vi "IVIDMM-Synchronized-Readout.vi"() -> ()   [LabVIEW 2015, in "IVI_DMM.lvlib"]
uses:
  IVI_DMM.lvlib
panel:
  in  "IVI Logical Names":refnum<k15>[](array[refnum])=["DMM3458A_GPIB0_21", "DMM3458A_GPIB0_22"]
  out "dt":dbl[unit] format="%.3f"
  out "Apertures":dbl[unit][](array[numeric])
  out "Samples":i32[](array[numeric])
  out "Graph":dbl[unit][](graph)
  in  "sample count":i32=10 caption="sample count (1)"
  in  "sample interval":dbl[unit]=0.1 caption="sample interval (0.0 s)" format="%.3f"
  out "error out":errorcluster
  in  "Stop":bool
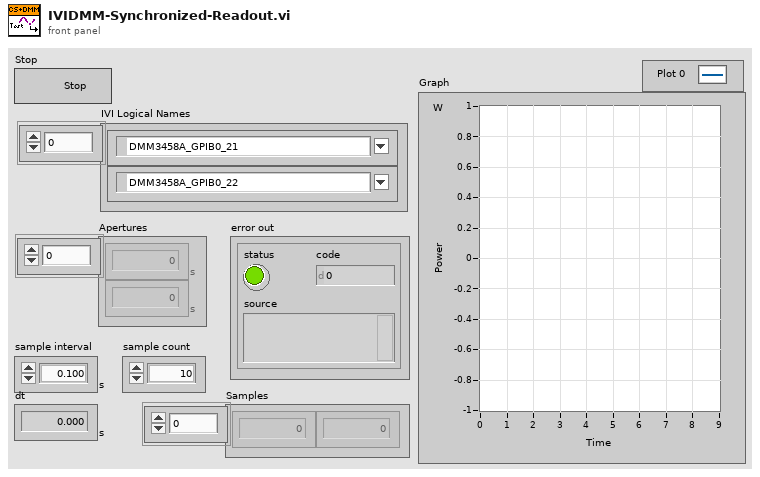
[diagram p1: front panel]
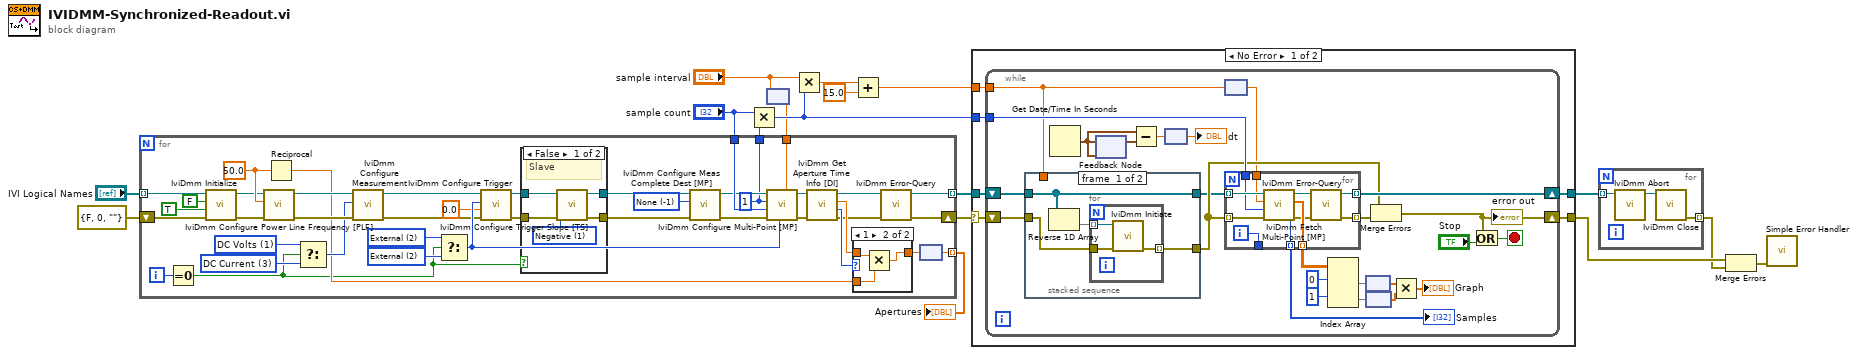
[diagram p0: block diagram]
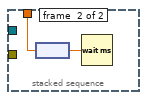
[diagram p2: hidden frame]
diagram:
  n1 = node("sample interval") -> (w3:dbl)
  n2 = for {
    tunnel: [w18] -> w17 mode=indexing
    shift-right: [w20] -> w16
    shift-left: errorcluster {"status"=FALSE, "code"=0, "source"=""} ("error out") -> [w26]
    tunnel: "sample count" -> [w48]
    tunnel: w3 -> [w47]
    tunnel: [w41] -> w8 mode=indexing
    tunnel: [w27] -> w7
    tunnel: "IVI Logical Names" -> [w24] mode=indexing
    i -> [w52]
    w49 = -1 items=["None"=-1, "External"=2, "PXI TRIG0 or VXI TTL0"=111, "PXI TRIG1 or VXI TTL1"=112, "PXI TRIG2 or VXI TTL2"=113, "PXI TRIG3 or VXI TTL3"=114, "PXI TRIG4 or VXI TTL4"=115, "PXI TRIG5 or VXI TTL5"=116, "PXI TRIG6 or VXI TTL6"=117, "PXI TRIG7 or VXI TTL7"=118, "ECL0"=119, "ECL1"=120, "PXI Star"=131, "RTSI 0"=140, "RTSI 1"=141, "RTSI 2"=142, "RTSI 3"=143, "RTSI 4"=144, "RTSI 5"=145, "RTSI 6"=146] ("meas complete dest (None)")
    w50 = 2 items=["Immediate"=1, "External"=2, "Software Trigger Function"=3, "Interval"=10, "PXI TRIG0 or VXI TTL0"=111, "PXI TRIG1 or VXI TTL1"=112, "PXI TRIG2 or VXI TTL2"=113, "PXI TRIG3 or VXI TTL3"=114, "PXI TRIG4 or VXI TTL4"=115, "PXI TRIG5 or VXI TTL5"=116, "PXI TRIG6 or VXI TTL6"=117, "PXI TRIG7 or VXI TTL7"=118, "ECL0"=119, "ECL1"=120, "PXI Star"=131, "RTSI 0"=140, "RTSI 1"=141, "RTSI 2"=142, "RTSI 3"=143, "RTSI 4"=144, "RTSI 5"=145, "RTSI 6"=146] ("sample trigger (Immediate)")
    w51 = 2 items=["Immediate"=1, "External"=2, "Software Trigger Function"=3, "Interval"=10, "PXI TRIG0 or VXI TTL0"=111, "PXI TRIG1 or VXI TTL1"=112, "PXI TRIG2 or VXI TTL2"=113, "PXI TRIG3 or VXI TTL3"=114, "PXI TRIG4 or VXI TTL4"=115, "PXI TRIG5 or VXI TTL5"=116, "PXI TRIG6 or VXI TTL6"=117, "PXI TRIG7 or VXI TTL7"=118, "ECL0"=119, "ECL1"=120, "PXI Star"=131, "RTSI 0"=140, "RTSI 1"=141, "RTSI 2"=142, "RTSI 3"=143, "RTSI 4"=144, "RTSI 5"=145, "RTSI 6"=146] ("sample trigger (Immediate)")
    w27 = 1 ("trigger count (1)")
    w53 = 3 items=["DC Volts"=1, "AC Volts"=2, "DC Current"=3, "AC Current"=4, "2 Wire Resistance"=5, "4 Wire Resistance"=101, "AC + DC Volts"=106, "AC + DC Current"=107, "Frequency"=104, "Period"=105, "Temperature"=108] ("measurement function (DC Volts)")
    w55 = 1 items=["DC Volts"=1, "AC Volts"=2, "DC Current"=3, "AC Current"=4, "2 Wire Resistance"=5, "4 Wire Resistance"=101, "AC + DC Volts"=106, "AC + DC Current"=107, "Frequency"=104, "Period"=105, "Temperature"=108] ("measurement function (DC Volts)")
    w43 = 50.0 ("power line frequency (60.0 Hz)")
    n3 = Equal To 0?(x=w52) -> (x = 0?=w38:bool)
    n4 = call <vilib>:"IviDmm Initialize.vi"("error in (no error)"=w26, "reset device (True)"=TRUE ("Reset (F)"), "id query (True)"=FALSE, "logical name (\"SampleDmm\")"=w24) -> ("error out"=w22:errorcluster, "instrument handle out"=w23:refnum<k15>)  [unwired: 6 in]
    n5 = call <vilib>:"IviDmm Configure Power Line Frequency [PLF].vi"("error in (no error)"=w22, "power line frequency (60.0 Hz)"=w43, "instrument handle"=w23) -> ("error out"=w56:errorcluster, "instrument handle out"=w57:refnum<k15>)  [unwired: 7 in]
    n6 = Reciprocal(x=w43) -> (1/x=w42:dbl)
    n7 = Select(t=w55, s=w38, f=w53) -> (s? t:f=w54:i32)
    n8 = call <vilib>:"IviDmm Configure Measurement.vi"("error in (no error)"=w56, "measurement function (DC Volts)"=w54, "instrument handle"=w57) -> ("error out"=w32:errorcluster, "instrument handle out"=w33:refnum<k15>)  [unwired: 7 in]
    n9 = Select(t=w51, s=w38, f=w50) -> (s? t:f=w35:i32)
    n10 = call <vilib>:"IviDmm Configure Trigger.vi"("error in (no error)"=w32, "trigger delay (0.0 s)"=0.0, "trigger source (Immediate)"=w35, "instrument handle"=w33) -> ("error out"=w36:errorcluster, "instrument handle out"=w37:refnum<k15>)  [unwired: 6 in]
    n11 = case shown="False" w38 {
      tunnel: w37 -> [w63 w65]
      tunnel: [w62 w65] -> w40
      tunnel: w36 -> [w61 w64]
      tunnel: [w60 w64] -> w39
      frame False {
        w59 = 1 items=["Positive", "Negative"] ("trigger slope (0: Positive)")
        # "Slave"
        n12 = call <vilib>:"IviDmm Configure Trigger Slope [TS].vi"("error in (no error)"=w61, "trigger slope (0: Positive)"=w59, "instrument handle"=w63) -> ("error out"=w60:errorcluster, "instrument handle out"=w62:refnum<k15>)  [unwired: 7 in]
      }
      frame True {
        # "Master"
      }
    }
    n13 = call <vilib>:"IviDmm Configure Meas Complete Dest [MP].vi"("error in (no error)"=w39, "meas complete dest (None)"=w49, "instrument handle"=w40) -> ("error out"=w30:errorcluster, "instrument handle out"=w31:refnum<k15>)  [unwired: 7 in]
    n14 = call <vilib>:"IviDmm Configure Multi-Point [MP].vi"("sample interval (0.0 s)"=w47, "sample trigger (Immediate)"=w35, "error in (no error)"=w30, "sample count (1)"=w48, "trigger count (1)"=w27, "instrument handle"=w31) -> ("error out"=w28:errorcluster, "instrument handle out"=w29:refnum<k15>)  [unwired: 4 in]
    n15 = call <vilib>:"IviDmm Get Aperture Time Info [DI].vi"("error in (no error)"=w28, "instrument handle"=w29) -> ("error out"=w21:errorcluster, "aperture time units"=w46:i32, "aperture time (sec)"=w45:dbl, "instrument handle out"=w19:refnum<k15>)  [unwired: 6 in]
    n16 = case shown="1" w46 {
      tunnel: w45 -> [w66 w69]
      tunnel: [w66 w67] -> w44
      tunnel: w42 -> [_ w68]
      frame 0, Default {
      }
      frame 1 {
        n17 = Multiply(x=w69, y=w68) -> (x*y=w67:dbl)
      }
    }
    n18 = call <vilib>:"IviDmm Error-Query.vi"("error in (no error)"=w21, "instrument handle"=w19) -> ("error out"=w20:errorcluster, "instrument handle out"=w18:refnum<k15>)  [unwired: 6 in, 2 out]
    n19 = node(w44) -> (w41:dbl[unit])
  }
  "Apertures" <- w8
  n20 = Multiply(x="sample count", y=w7) -> (x*y=w5:i32)
  n21 = Multiply(x="sample interval", y=w5) -> (x*y=w11:dbl[unit])
  n22 = Add(x=w11, y=dbl[unit] 15.0 ("x")) -> (x+y=w9:dbl[unit])
  n23 = case shown="No Error" w16 {
    selector: w16 -> [w74 w121]
    tunnel: w17 -> [w75 w122]
    tunnel: [w73 w122] -> w15
    tunnel: [w72 w121] -> w14
    tunnel: w9 -> [w71 _]
    tunnel: w5 -> [w70 _]
    frame No Error {
      n24 = while {
        shift-right: [w82] -> w72
        shift-left: w74 -> [w100]
        shift-right: [w98] -> w73
        shift-left: w75 -> [w97]
        tunnel: w71 -> [w77]
        tunnel: w70 -> [w96]
        stop <- w89 stop-if-true
        n25 = stacked-sequence {
          tunnel: w100 -> [w104 _]
          tunnel: w97 -> [w103 _]
          tunnel: [w101 _] -> w81
          tunnel: w77 -> [_ w108]
          tunnel: [w103 _] -> w76
          frame #0 {
            n26 = Reverse 1D Array(array=w103) -> (reversed array=w102:refnum<k15>[])
            n27 = for {
              tunnel: w102 -> [w105] mode=indexing
              tunnel: w104 -> [w107]
              tunnel: [w106] -> w101 mode=indexing
              n28 = call <vilib>:"IviDmm Initiate.vi"("error in (no error)"=w107, "instrument handle"=w105) -> ("error out"=w106:errorcluster)  [unwired: 8 in, 1 out]
            }
          }
          frame #1 {
            n29 = node(w108) -> (w109:dbl)
            n30 = Wait (ms)(milliseconds to wait=w109) -> ()  [unwired: 1 out]
          }
        }
        n31 = Get Date/Time In Seconds() -> (seconds since 1Jan1904=w86:timestamp)
        n32 = feedback #1(w86) -> (w85:timestamp)
        n33 = feedback-in #1(w86) -> ()
        n34 = Subtract(x=w86, y=w85) -> (x-y=w84:dbl)
        n35 = node(w84) -> (→"dt":dbl[unit])
        n36 = node(w77) -> (w78:dbl)
        n37 = for {
          tunnel: w76 -> [w119] mode=indexing
          tunnel: [w112] -> w98 mode=indexing
          tunnel: [w120] -> _
          tunnel: w96 -> [w117]
          tunnel: [w116] -> w95 mode=indexing
          tunnel: [w115] -> w87 mode=indexing
          tunnel: w78 -> [w113]
          tunnel: [w111] -> w88 mode=indexing
          tunnel: w81 -> [w114] mode=indexing
          i -> [w120]
          n38 = call <vilib>:"IviDmm Fetch Multi-Point [MP].vi"("error in (no error)"=w114, "array size (1)"=w117, "maximum time (5000 ms)"=w113, "instrument handle"=w119) -> ("error out"=w110:errorcluster, "actual number of points"=w115:i32, "reading array"=w116:dbl[], "instrument handle out"=w118:refnum<k15>)  [unwired: 4 in]
          n39 = call <vilib>:"IviDmm Error-Query.vi"("error in (no error)"=w110, "instrument handle"=w118) -> ("error out"=w111:errorcluster, "instrument handle out"=w112:refnum<k15>)  [unwired: 6 in, 2 out]
        }
        "Samples" <- w87
        n40 = Index Array(array=w95, index (row) #1=0 ("index (row)"), index (row) #2=1 ("index (row)")) -> (element #1=w92:dbl[], element #2=w91:dbl[])  [unwired: 2 in]
        n41 = node(w92) -> (w80:dbl[unit][])
        n42 = node(w91) -> (w79:dbl[unit][])
        n43 = Merge Errors(w81, w88) -> (w82:errorcluster)
        "error out" <- w82
        n44 = Multiply(x=w80, y=w79) -> (x*y=→"Graph":dbl[unit][])
        n45 = Or(x=w82, y="Stop") -> (x .or. y?=w89:bool)
      }
    }
    frame Error {
    }
  }
  n46 = for {
    tunnel: w15 -> [w125] mode=indexing
    tunnel: [w124] -> w13 mode=indexing
    n47 = call <vilib>:"IviDmm Abort.vi"("instrument handle"=w125) -> ("instrument handle out"=w123:refnum<k15>)  [unwired: 9 in, 1 out]
    n48 = call <vilib>:"IviDmm Close.vi"("instrument handle"=w123) -> ("error out"=w124:errorcluster)  [unwired: 10 in]
  }
  n49 = Merge Errors(w14, w13) -> (w12:errorcluster)
  n50 = call <vilib>:"Simple Error Handler.vi"("error in (no error)"=w12) -> ()  [unwired: 4 in, 5 out]
